vi "Handle Event.vi"(8 "error in (no error)":errorcluster, 9 "Event Source in":refnum<class "Event Source.lvclass">, 10 "Event Data":refnum<class "Event.lvclass">, 11 "Abstract Source Event Handler in":refnum<class "Abstract Source Event Handler.lvclass">) -> (0 "error out":errorcluster, 1 "Event Source out":refnum<class "Event Source.lvclass">, 3 "Abstract Source Event Handler out":refnum<class "Abstract Source Event Handler.lvclass">)   [LabVIEW 2016, in "Event Source.lvlib" / "Abstract Source Event Handler.lvclass"]
uses:
  Abstract Source Event Handler.lvclass
  Event/Event.lvclass
  Event Source/Event Source.lvclass
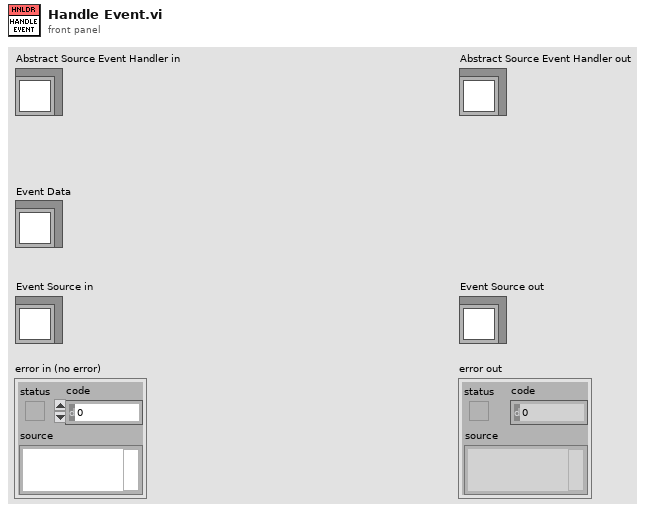
[diagram p1: front panel]
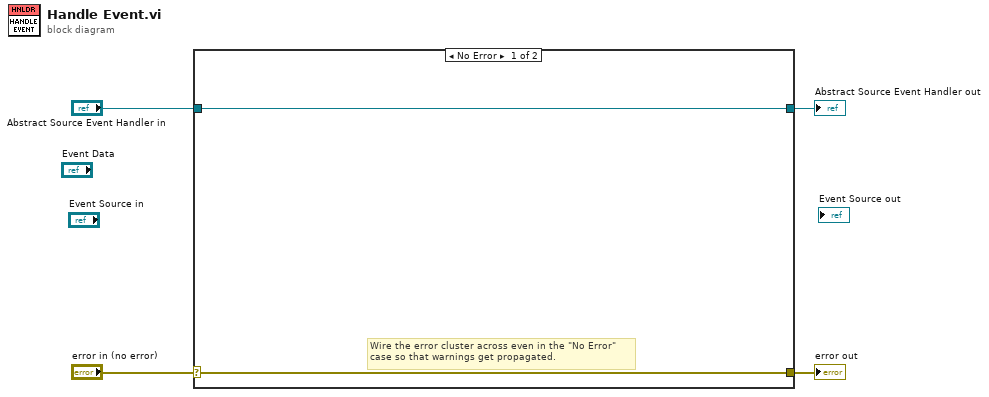
[diagram p0: block diagram]
diagram:
  n1 = case shown="No Error" "error in (no error)" {
    selector: "error in (no error)" -> [w5 w8]
    tunnel: [w5 w8] -> w3
    tunnel: [w6 w7] -> w1
    tunnel: "Abstract Source Event Handler in" -> [w6 w7]
    frame No Error {
      # "Wire the error cluster across even in the \"No Error\"\ncase so that warnings get propagated."
    }
    frame Error {
    }
  }
  "error out" <- w3
  "Abstract Source Event Handler out" <- w1
